vi "Test set cell font bold.vi"(11 "Test Case In":refnum<class "Test Cases.lvclass">) -> (0 "error out":errorcluster, 3 "Test Case Out":refnum<class "Test Cases.lvclass">)   [LabVIEW 2023, in "Test Cases.lvclass"]
uses:
  Test Cases.lvclass
  C:/Program Files/National Instruments/LabVIEW 2025/vi.lib/Astemes/LUnit/Test Case.lvclass
  D:/git/Sourcegrid-LabVIEW/dll/SourceGrid.dll
  dll/SourceGrid.dll
  source/Grid/SourceGrid.lvclass
  source/Cells/Cell/Cell.lvclass
  source/Views/Cell View/Cell View.lvclass
  <vilib>/Astemes/LUnit/Test Case.lvclass/Test Case.ctl
  <vilib>/Astemes/LUnit/Append Pass Result.vi
  <vilib>/Astemes/LUnit/Append Fail Result.vi
  <vilib>/Astemes/LUnit/Run In UI.vi
  <vilib>/Utility/error.llb/Clear Errors.vi
  source/Grid/Set Column Default Width.vi
  source/Font/Font.lvclass
  <vilib>/Astemes/LUnit/Test Case.lvclass
panel:
  in  "stop":bool
  in  "Grid Container":refnum<k24>(container)
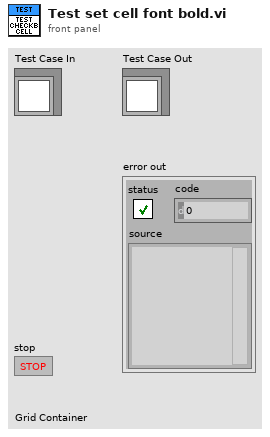
[diagram p1: front panel]
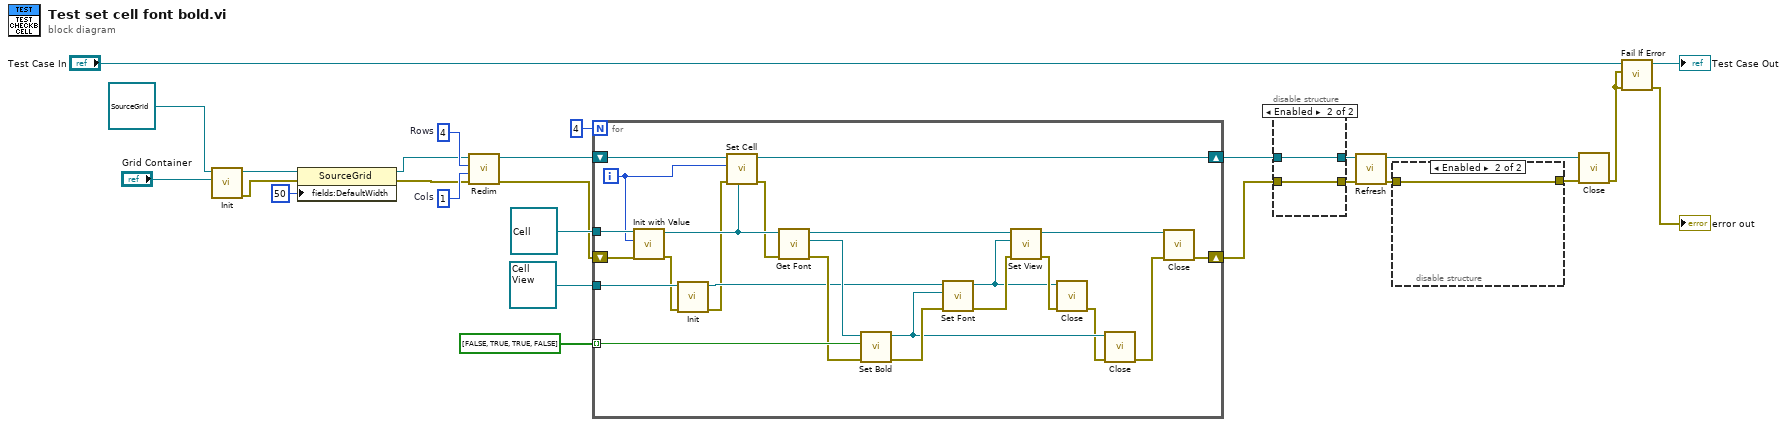
[diagram p0: block diagram]
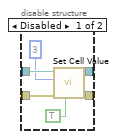
[diagram p2: hidden frame]
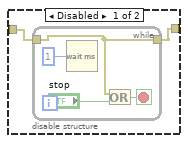
[diagram p3: hidden frame]
diagram:
  w22 = 1  # Cols
  w23 = 4  # Rows
  n1 = call-dynamic "Init.vi"("Sourcegrid Container"="Grid Container", "Grid in"=refnum<class "SourceGrid.lvclass"> refnum) -> ("error out"=w12:errorcluster, "Grid out"=w19:refnum<class "SourceGrid.lvclass">)  [unwired: 8 in]
  n2 = property class="SourceGrid"(reference=w19, error in=w12, "fields:DefaultWidth"=50 ("DefaultWidth")) -> (reference out=w18:refnum<class "SourceGrid.lvclass">, error out=w17:errorcluster)
  n3 = call "Redim.vi"("error in"=w17, "Columns"=w22, "Rows"=w23, "Sourcegrid in"=w18) -> ("error out"=w7:errorcluster, "Sourcegrid out"=w15:refnum<class "SourceGrid.lvclass">)  [unwired: 6 in]
  n4 = for {
    N: 4 -> [_]
    shift-right: [w49] -> w8
    shift-left: w7 -> [w36]
    shift-right: [w42] -> w5
    shift-left: w15 -> [w50]
    tunnel: refnum<class "Cell.lvclass"> refnum ("Cell in") -> [w48]
    tunnel: bool[] [FALSE, TRUE, TRUE, FALSE] -> [w46] mode=indexing
    tunnel: refnum<class "Cell View.lvclass"> refnum ("SourceGrid.lvlib:Cell View.lvclass") -> [w37]
    i -> [w47]
    n5 = call-dynamic "Init with Value.vi"("error in"=w36, "Value"=w47, "Cell in"=w48) -> ("error out"=w35:errorcluster, "Cell out"=w44:refnum<class "Cell.lvclass">)  [unwired: 7 in]
    n6 = call-dynamic "Init.vi"("error in"=w35, "Cell View in"=w37) -> ("error out"=w30:errorcluster, "Cell View out"=w34:refnum<class "Cell View.lvclass">)  [unwired: 8 in]
    n7 = call "Set Cell.vi"("Cell"=w44, "error in"=w30, "Row"=w47, "Sourcegrid in"=w50) -> ("error out"=w43:errorcluster, "Sourcegrid out"=w42:refnum<class "SourceGrid.lvclass">)  [unwired: 6 in]
    n8 = call-dynamic "Get Font.vi"("error in"=w43, "Cell in"=w44) -> ("error out"=w39:errorcluster, "Font out"=w38:refnum<class "Font.lvclass">, "Cell out"=w40:refnum<class "Cell.lvclass">)  [unwired: 7 in]
    n9 = call "Set Bold.vi"("error in"=w39, "Bold"=w46, "Font in"=w38) -> ("error out"=w33:errorcluster, "Font out"=w31:refnum<class "Font.lvclass">)  [unwired: 7 in]
    n10 = call-dynamic "Set Font.vi"("error in"=w33, "Font.lvclass"=w31, "View in"=w34) -> ("error out"=w32:errorcluster, "View out"=w28:refnum<class "Cell View.lvclass">)  [unwired: 7 in]
    n11 = call-dynamic "Set View.vi"("error in"=w32, "CellView"=w28, "Cell in"=w40) -> ("error out"=w29:errorcluster, "Cell out"=w41:refnum<class "Cell.lvclass">)  [unwired: 7 in]
    n12 = call-dynamic "Close.vi"("error in"=w29, "Cell View in"=w28) -> ("error out"=w27:errorcluster)  [unwired: 8 in, 1 out]
    n13 = call-dynamic "Close.vi"("error in"=w27, "Font in"=w31) -> ("error out"=w45:errorcluster)  [unwired: 8 in, 1 out]
    n14 = call-dynamic "Close.vi"("error in"=w45, "Cell in"=w41) -> ("error out"=w49:errorcluster)  [unwired: 8 in, 1 out]
  }
  n15 = disable-structure shown="Enabled" {
    disable-tunnel: w8 -> [w56 w57]
    disable-tunnel: [w55 w57] -> w6
    disable-tunnel: w5 -> [w54 w58]
    disable-tunnel: [w53 w58] -> w4
    frame Disabled {
      n16 = call "Set Cell Value.vi"("Value"=TRUE, "error in"=w56, "Row"=3, "SourceGrid in"=w54) -> ("error out"=w55:errorcluster, "SourceGrid out"=w53:refnum<class "SourceGrid.lvclass">)  [unwired: 6 in]
    }
    frame Enabled {
    }
  }
  n17 = call "Refresh.vi"("error in"=w6, "SourceGrid in"=w4) -> ("error out"=w10:errorcluster, "SourceGrid out"=w13:refnum<class "SourceGrid.lvclass">)  [unwired: 8 in]
  n18 = disable-structure shown="Enabled" {
    disable-tunnel: w10 -> [w60 w65]
    disable-tunnel: [w59 w65] -> w9
    frame Disabled {
      n19 = while {
        tunnel: w60 -> [w61]
        tunnel: [w61] -> w59
        stop <- w62 stop-if-true
        n20 = Wait (ms)(milliseconds to wait=u32 1) -> ()  [unwired: 1 out]
        n21 = Or(x=w61, y="stop") -> (x .or. y?=w62:bool)
      }
    }
    frame Enabled {
    }
  }
  n22 = call-dynamic "Close.vi"("error in"=w9, "Sourcegrid in"=w13) -> ("error out"=w21:errorcluster)  [unwired: 8 in, 1 out]
  n23 = call <vilib>:"Fail If Error.vi"("error in (no error)"=w21, "Assert error"=w21, "LUnit Test Case In"="Test Case In") -> ("error out"=→"error out":errorcluster, "LUnit Test Case Out"=→"Test Case Out":refnum<class "Test Cases.lvclass">)  [unwired: 7 in]
